vi "State_Machine.vi"() -> ()   [LabVIEW 2020, in "State_Machine_Queue.lvlib"]
doc: "Simple string based state machine."
uses:
  State_Machine_Queue.lvlib
  <vilib>/Utility/error.llb/Error Cluster From Error Code.vi
  <vilib>/ErrorRing/Error Ring.xnode
panel:
  out "Error Out":errorcluster
  in  "Error In":errorcluster
  out "Reply":string
  in  "Ultimate Question":bool
  in  "Ultimate Answer":bool
  in  "Stop":bool
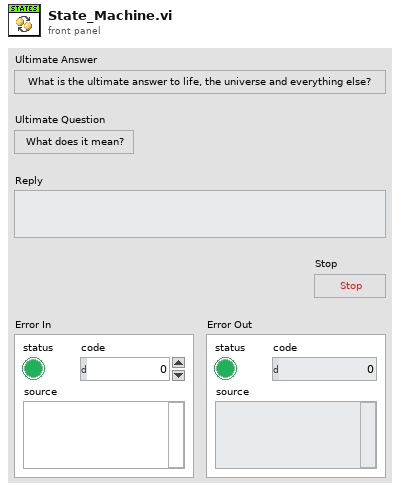
[diagram p1: front panel]
types:
  T1 = enum16{"Obtain", "Enqueue", "Get Queue", "Flush", "Release"}
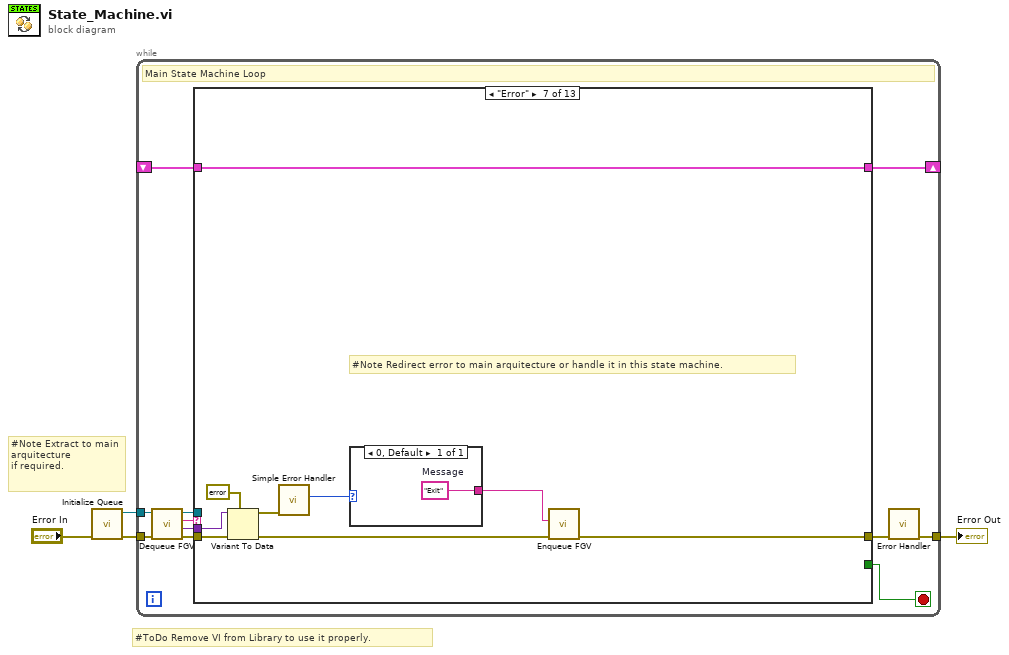
[diagram p0: block diagram]
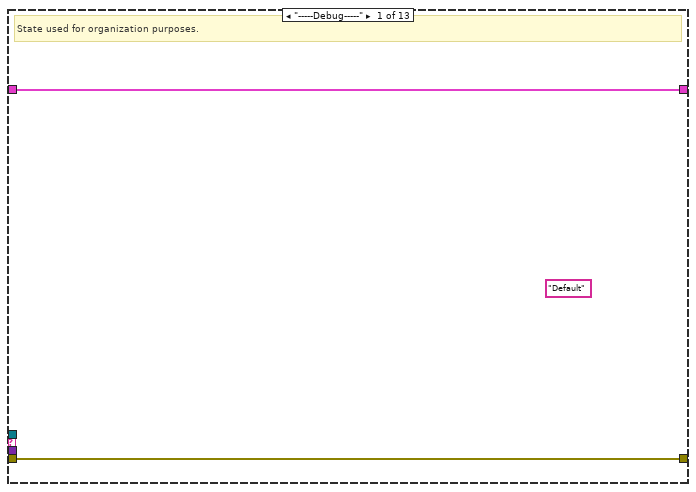
[diagram p2: hidden frame]
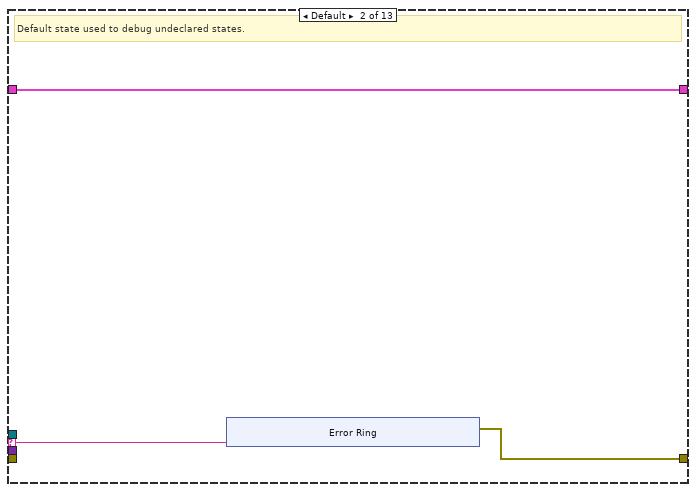
[diagram p3: hidden frame]
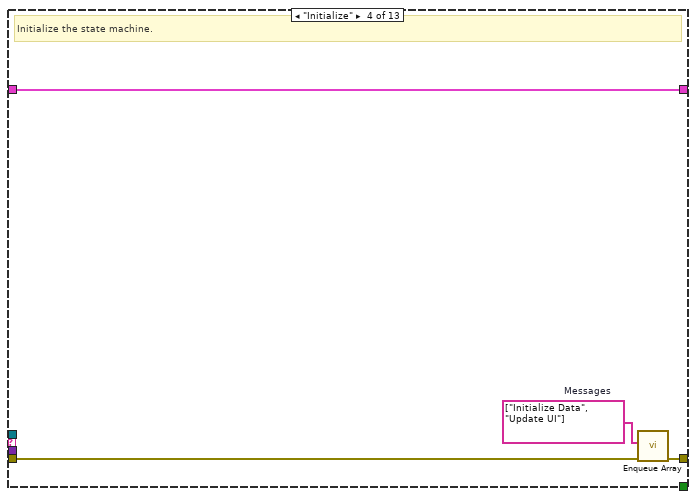
[diagram p5: hidden frame]
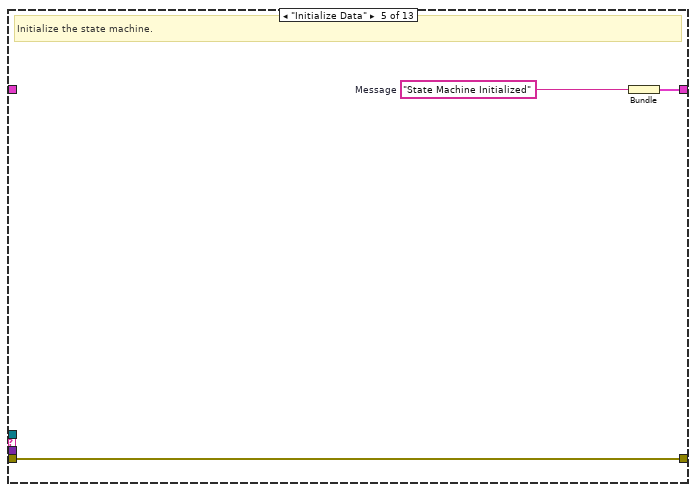
[diagram p6: hidden frame]
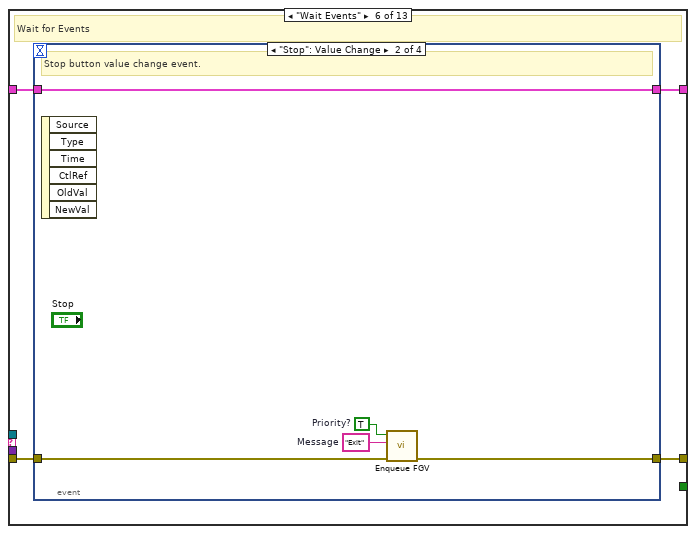
[diagram p7: hidden frame]
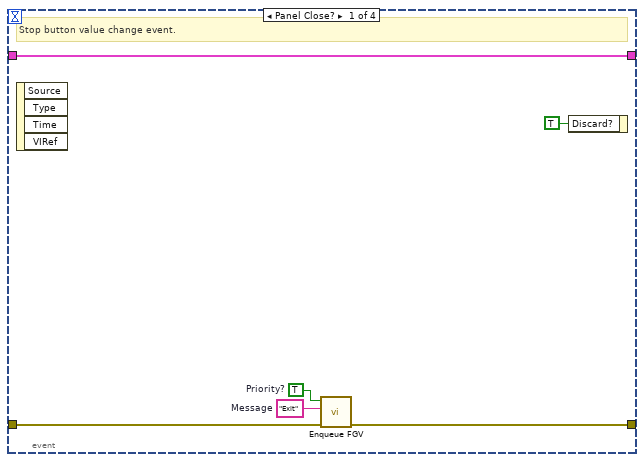
[diagram p8: hidden frame]
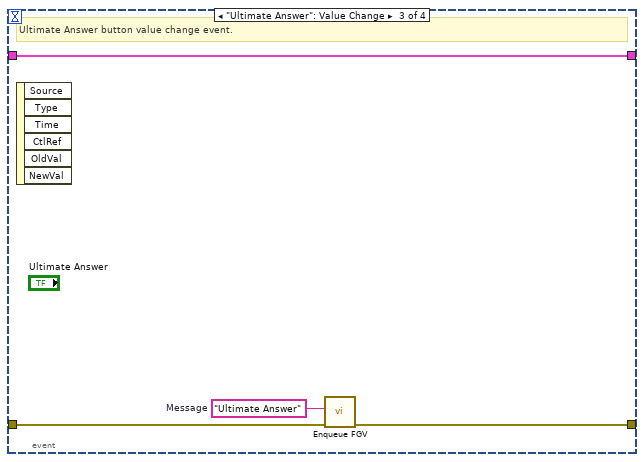
[diagram p9: hidden frame]
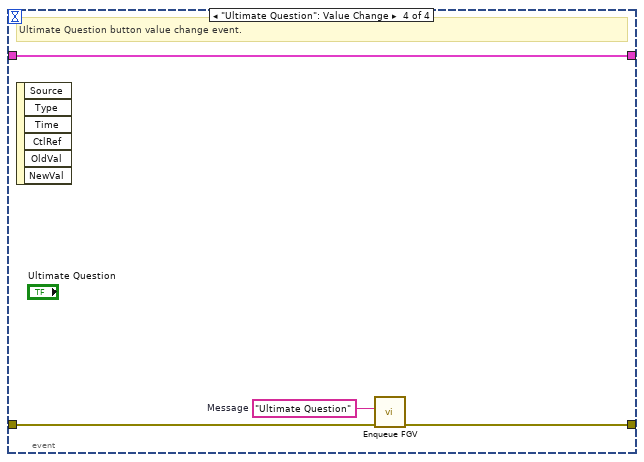
[diagram p10: hidden frame]
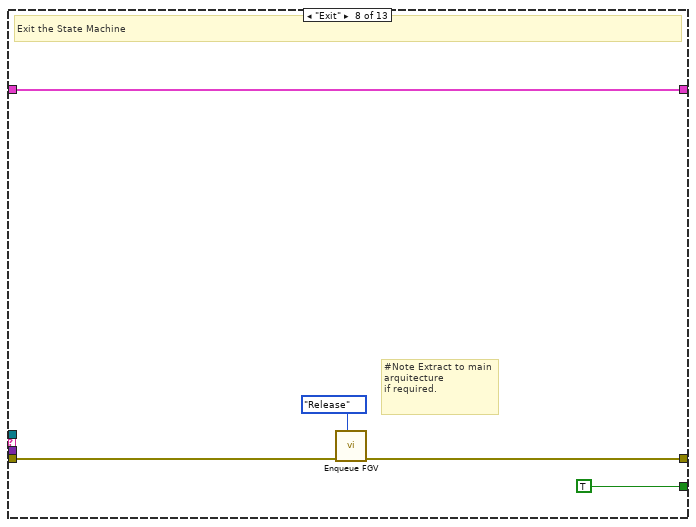
[diagram p11: hidden frame]
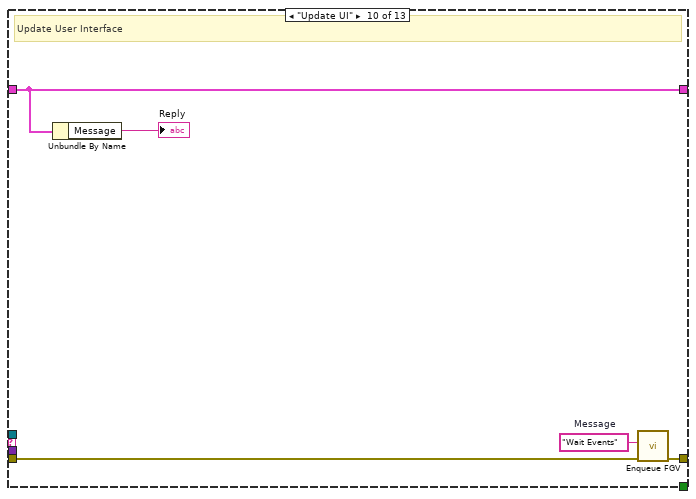
[diagram p13: hidden frame]
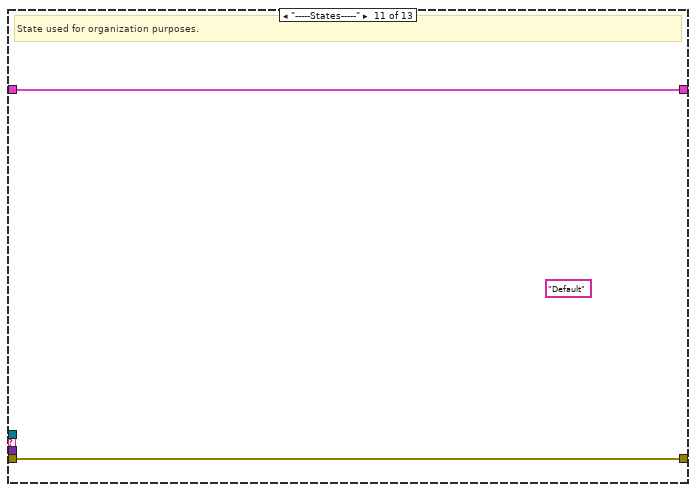
[diagram p14: hidden frame]
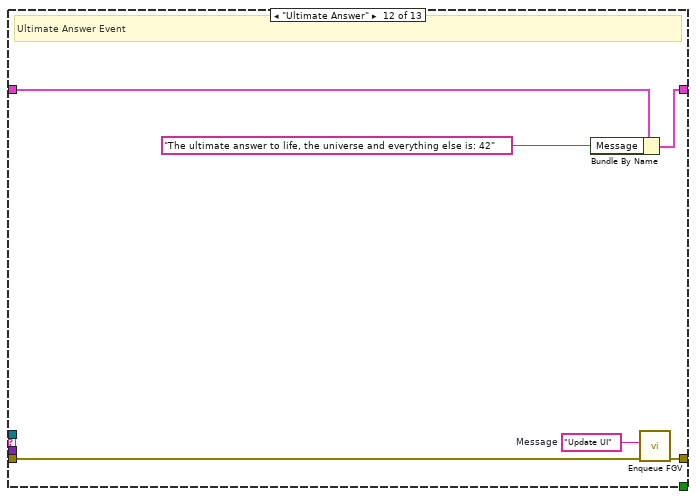
[diagram p15: hidden frame]
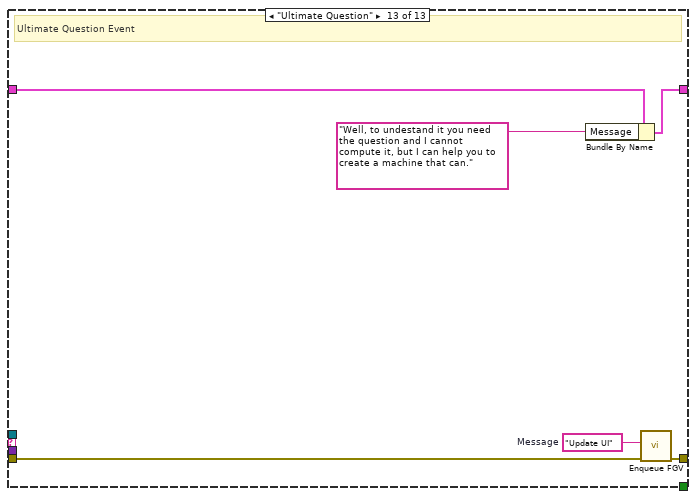
[diagram p16: hidden frame]
diagram:
  # "#ToDo Remove VI from Library to use it properly."
  # "#Note Extract to main arquitecture\nif required."
  n1 = call "Initialize Queue.vi"("error in"="Error In") -> ("error out"=w1:errorcluster, "Queue out"=w2:refnum<queue>)  [unwired: 9 in]
  n2 = while {
    shift-right: [w14] -> _
    shift-left: _ -> [w15]
    tunnel: w1 -> [w12]
    tunnel: [w10] -> w4
    tunnel: w2 -> [w5]
    stop <- w13 stop-if-true
    # "Main State Machine Loop"
    n3 = call "Dequeue FGV.vi"("error in"=w12, "queue in"=w5) -> ("error out"=w11:errorcluster, "Message Data"=w7:variant, "Message"=w8:string, "queue out"=w6:refnum<queue>)  [unwired: 6 in]
    n4 = case shown="\"Error\"" w8 {
      selector: w8 -> [_ w19 _ _ _ _ _ _ _ _ _ _ _]
      tunnel: w11 -> [w17 _ w29 w32 w34 w40 w67 w71 w76 w78 w83 w84 w90]
      tunnel: [w17 w18 w29 w33 w34 w39 w62 w72 w76 w79 w83 w85 w91] -> w9
      tunnel: [_ _ _ _ _ _ _ TRUE _ _ _ _ _] -> w13
      tunnel: w15 -> [w16 w20 w28 w30 _ w38 w68 w73 w75 w81 w82 w89 w95]
      tunnel: [w16 w20 w28 w30 w35 w37 w68 w73 w75 w81 w82 w88 w94] -> w14
      tunnel: w7 -> [_ _ _ _ _ _ w66 _ _ _ _ _ _]
      tunnel: w6 -> [_ _ _ _ _ _ _ _ _ _ _ _ _]
      frame "-----Debug-----" {
        (unwired) "Default" ("State")
        # "State used for organization purposes."
      }
      frame Default {
        # "Default state used to debug undeclared states."
        n5 = xnode "Error Ring"("parameter 0"=w19) -> ("error out"=w18:errorcluster)
      }
      frame "-----Core-----" {
        # "State used for organization purposes."
      }
      frame "Initialize" {
        w31 = string[] ["Initialize Data", "Update UI"]  # Messages
        # "Initialize the state machine."
        n6 = call "Enqueue Array.vi"("error in"=w32, "Messages"=w31) -> ("error out"=w33:errorcluster)  [unwired: 9 in]
      }
      frame "Initialize Data" {
        w36 = "State Machine Initialized"  # Message
        # "Initialize the state machine."
        n7 = Bundle("Message"=w36) -> (w35:cluster{"Message":string})  [unwired: 1 in]
      }
      frame "Wait Events" {
        # "Wait for Events"
        n8 = event shown="[1] \"Stop\": Value Change" {
          selector: _ -> [_ _ _ _]
          dyn-events: _ -> [_ _ _ _]
          timeout: _ -> [_ _ _ _]
          tunnel: w40 -> [w43 w48 w53 w57]
          tunnel: [w44 w47 w52 w56] -> w39
          tunnel: w38 -> [w46 w51 w55 w59]
          tunnel: [w46 w51 w55 w59] -> w37
          event Panel Close? {
            w41 = "Exit"  # Message
            w42 = TRUE  # Priority?
            # "Stop button value change event."
            n9 = event-data() -> ()  [unwired: 1 in, 4 out]
            n10 = call "Enqueue FGV.vi"("error in"=w43, "Message"=w41, "Priority?"=w42) -> ("error out"=w44:errorcluster)  [unwired: 7 in, 1 out]
            n11 = event-data("Discard?"=TRUE) -> ()  [unwired: 1 in, 1 out]
          }
          event "Stop": Value Change {
            w49 = "Exit"  # Message
            w50 = TRUE  # Priority?
            # "Stop button value change event."
            n12 = event-data() -> ()  [unwired: 1 in, 6 out]
            n13 = call "Enqueue FGV.vi"("error in"=w48, "Message"=w49, "Priority?"=w50) -> ("error out"=w47:errorcluster)  [unwired: 7 in, 1 out]
          }
          event "Ultimate Answer": Value Change {
            w54 = "Ultimate Answer"  # Message
            # "Ultimate Answer button value change event."
            n14 = event-data() -> ()  [unwired: 1 in, 6 out]
            n15 = call "Enqueue FGV.vi"("error in"=w53, "Message"=w54) -> ("error out"=w52:errorcluster)  [unwired: 8 in, 1 out]
          }
          event "Ultimate Question": Value Change {
            w58 = "Ultimate Question"  # Message
            # "Ultimate Question button value change event."
            n16 = event-data() -> ()  [unwired: 1 in, 6 out]
            n17 = call "Enqueue FGV.vi"("error in"=w57, "Message"=w58) -> ("error out"=w56:errorcluster)  [unwired: 8 in, 1 out]
          }
        }
      }
      frame "Error" {
        # "#Note Redirect error to main arquitecture or handle it in this state machine."
        n18 = Variant To Data(error in=w67, type=errorcluster {"status"=FALSE, "code"=0, "source"=""} ("error constant"), Variant=w66) -> (data=w64:errorcluster, error out=w63:errorcluster)
        n19 = call <vilib>:"Simple Error Handler.vi"("error in (no error)"=w64) -> ("code out"=w61:i32)  [unwired: 4 in, 4 out]
        n20 = case shown="0, Default" w61 {
          tunnel: [w69] -> w60
          frame 0, Default {
            w69 = "Exit"  # Message
          }
        }
        n21 = call "Enqueue FGV.vi"("error in"=w63, "Message"=w60) -> ("error out"=w62:errorcluster)  [unwired: 8 in, 1 out]
      }
      frame "Exit" {
        # "#Note Extract to main arquitecture\nif required."
        # "Exit the State Machine"
        n22 = call "Enqueue FGV.vi"("Actions"=T1."Release", "error in"=w71) -> ("error out"=w72:errorcluster)  [unwired: 8 in, 1 out]
      }
      frame "-----User Interface-----" {
        # "State used for organization purposes."
      }
      frame "Update UI" {
        w77 = "Wait Events"  # Message
        # "Update User Interface"
        n23 = Unbundle By Name(w81) -> ("Message"=→"Reply":string)
        n24 = call "Enqueue FGV.vi"("error in"=w78, "Message"=w77) -> ("error out"=w79:errorcluster)  [unwired: 8 in, 1 out]
      }
      frame "-----States-----" {
        (unwired) "Default" ("State")
        # "State used for organization purposes."
      }
      frame "Ultimate Answer" {
        w86 = "Update UI"  # Message
        # "Ultimate Answer Event"
        n25 = Bundle By Name(cluster=w89, "Message"="The ultimate answer to life, the universe and everything else is: 42") -> (w88:cluster{"Message":string})
        n26 = call "Enqueue FGV.vi"("error in"=w84, "Message"=w86) -> ("error out"=w85:errorcluster)  [unwired: 8 in, 1 out]
      }
      frame "Ultimate Question" {
        w92 = "Update UI"  # Message
        # "Ultimate Question Event"
        n27 = Bundle By Name(cluster=w95, "Message"="Well, to undestand it you need the question and I cannot compute it, but I can help you to create a machine that can.") -> (w94:cluster{"Message":string})
        n28 = call "Enqueue FGV.vi"("error in"=w90, "Message"=w92) -> ("error out"=w91:errorcluster)  [unwired: 8 in, 1 out]
      }
    }
    n29 = call "Error Handler.vi"("error in"=w9) -> ("dup error in"=w10:errorcluster)  [unwired: 9 in, 1 out]
  }
  "Error Out" <- w4
